vi "FPGA_PPG_query_mode.vi"(0 "resource_in":refnum<visa-resource-name>, 5 "error in (no error)":errorcluster) -> (14 "resource_out":refnum<visa-resource-name>, 16 "mode":i16, 19 "error out":errorcluster)   [LabVIEW 2014, in "NI-FPGA_PPG_Driver.lvlib"]
doc: "Queries the execution mode of the FPGA.\n\nContact: Falk Ziegler, eMail: ziegler@physik.uni-greifswald.de"
uses:
  NI-FPGA_PPG_Driver.lvlib
  <vilib>/rvi/interface/nirviReadWriteControl/nirviReadWriteControl.xnode
  FPGA_PPG_action_type.ctl
  FPGA_PPG_vi_ref.ctl
  D:/Workspace/PyCharm/Tilda/TildaTarget/Labview14/FPGA Bitfiles/TiTaProj_COF_PPG_100MHz.lvbitx
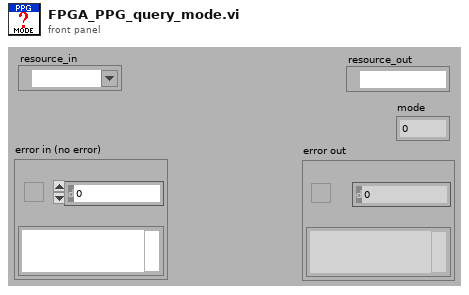
[diagram p1: front panel]
types:
  T1 = typedef "NI-FPGA_PPG_Driver.lvlib/FPGA_PPG_action_type.ctl" = enum16{"GET", "SET", "REMOVE"}
  T2 = typedef "NI-FPGA_PPG_Driver.lvlib/FPGA_PPG_vi_ref.ctl" = refnum<k20>
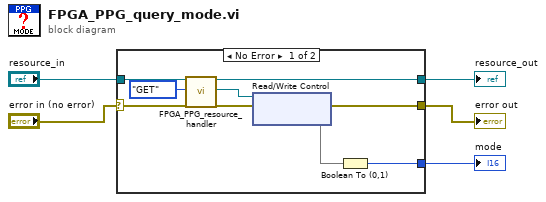
[diagram p0: block diagram]
diagram:
  n1 = case shown="No Error" "error in (no error)" {
    selector: "error in (no error)" -> [w13 w16]
    tunnel: [w8 w16] -> w4
    tunnel: "resource_in" -> [w14 w15]
    tunnel: [w9 w15] -> w2
    tunnel: [w10 _] -> w1
    frame No Error {
      n2 = call "FPGA_PPG_resource_handler.vi"("resource_in"=w14, "action"=FPGA_PPG_action_type."GET", "error in (no error)"=w13) -> ("resource_out"=w9:refnum<visa-resource-name>, "FPGA VI Reference Out"=w7:T2, "error out"=w12:errorcluster)  [unwired: 14 in]
      n3 = xnode "Read/Write Control"("FPGA VI Reference In"=w7, "error in"=w12) -> ("error out"=w8:errorcluster, "continuous"=w11)  [unwired: 1 out]
      n4 = Boolean To (0,1)(Boolean=w11) -> (0, 1=w10:i16)
    }
    frame Error {
    }
  }
  "error out" <- w4
  "resource_out" <- w2
  "mode" <- w1
